vi "UT_EField_DAQ_AnalogIO.ProcPeriodic.vi"(0 "i ref in":refnum<vi>, 3 "ms timeout (10000)":i32=10000, 5 "error in (no error)":errorcluster) -> (14 "i ref out":refnum<vi>, 17 "timed out":bool, 19 "error out":errorcluster)   [LabVIEW 2014, in "UT_EField_DAQ_AnalogIO.lvlib"]
doc: "This method serves to periodically do things like reading values from the HW. Methods that should be executed periodically should be called from THIS methode. Add code here."
uses:
  UT_EField_DAQ_AnalogIO.lvlib
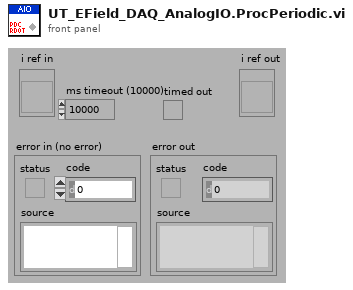
[diagram p1: front panel]
types:
  T1 = typedef "UT_EField_DAQ_AnalogIO.lvlib/UT_EField_DAQ_AnalogIO.i attribute.ctl" = cluster{"inputs":cluster{"index":i32[], "channel_task":refnum<k21>[], "range":cluster{"min":dbl, "max":dbl}[], "channel_number":i32, "scale_factor":dbl}, "outputs":cluster{"index":i32[], "channel_task":refnum<k21>[], "range":cluster{"min":dbl, "max":dbl}[], "channel_number":i32, "scale_factor":dbl}}
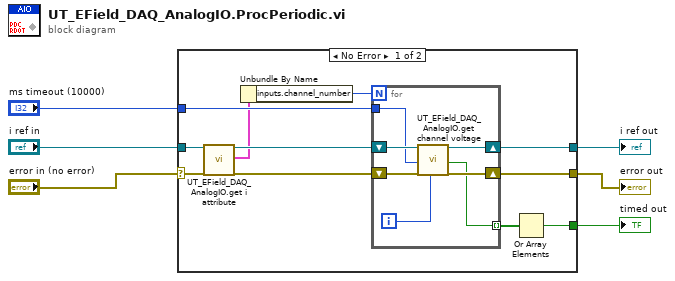
[diagram p0: block diagram]
diagram:
  n1 = case shown="No Error" "error in (no error)" {
    selector: "error in (no error)" -> [w16 w25]
    tunnel: "i ref in" -> [w17 w26]
    tunnel: [w13 w26] -> w4
    tunnel: [w12 w25] -> w3
    tunnel: "ms timeout (10000)" -> [w11 _]
    tunnel: [w9 _] -> w1
    frame No Error {
      n2 = call "UT_EField_DAQ_AnalogIO.get i attribute.vi"("i ref in"=w17, "error in (no error)"=w16) -> ("i ref out"=w15:refnum<vi>, "i attribute"=w8:T1, "error out"=w14:errorcluster)  [unwired: 15 in]
      n3 = Unbundle By Name(w8) -> ("inputs.channel_number"=w7:i32)
      n4 = for {
        N: w7 -> [_]
        shift-right: [w22] -> w13
        shift-left: w15 -> [w24]
        shift-right: [w21] -> w12
        shift-left: w14 -> [w23]
        tunnel: w11 -> [w19]
        tunnel: [w18] -> w10 mode=indexing
        i -> [w20]
        n5 = call "UT_EField_DAQ_AnalogIO.get channel voltage.vi"("i ref in"=w24, "Timeout"=w19, "error in"=w23, "channel_index"=w20) -> ("i ref out"=w22:refnum<vi>, "timed out"=w18:bool, "error out"=w21:errorcluster)  [unwired: 12 in, 1 out]
      }
      n6 = Or Array Elements(Boolean array=w10) -> (logical OR=w9:bool)
    }
    frame Error {
    }
  }
  "error out" <- w3
  "i ref out" <- w4
  "timed out" <- w1
